vi "ProgInit.vi"(3 "error in (no error)":errorcluster, 4 "Intialize?":bool, 5 "EpiWrapper in":refnum<class "EpiWrapper.lvclass">) -> (0 "error out":errorcluster, 2 "EpiWrapper out":refnum<class "EpiWrapper.lvclass">)   [LabVIEW 2012, in "EpiWrapper.lvclass"]
uses:
  EpiWrapper.lvclass
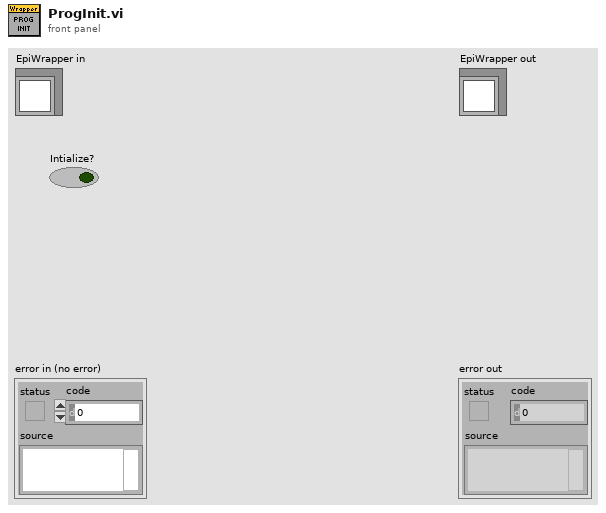
[diagram p1: front panel]
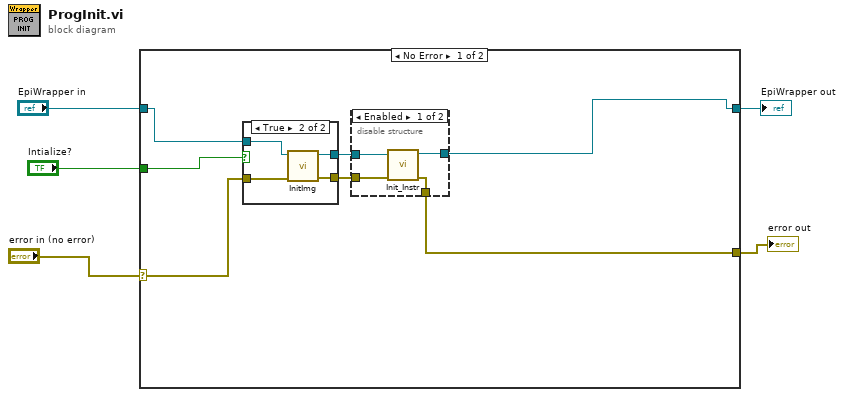
[diagram p0: block diagram]
diagram:
  n1 = case shown="No Error" "error in (no error)" {
    selector: "error in (no error)" -> [w6 w26]
    tunnel: [w9 w26] -> w4
    tunnel: [w10 w25] -> w2
    tunnel: "EpiWrapper in" -> [w7 w25]
    tunnel: "Intialize?" -> [w8 _]
    frame No Error {
      n2 = case shown="True" w8 {
        tunnel: [w14 w18] -> w12
        tunnel: [w13 w17] -> w11
        tunnel: w7 -> [w14 w16]
        tunnel: w6 -> [w13 w15]
        frame False {
        }
        frame True {
          n3 = call-dynamic "InitImg.vi"("error in (no error)"=w15, "EpiWrapper in"=w16) -> ("error out"=w17:errorcluster, "EpiWrapper out"=w18:refnum<class "EpiWrapper.lvclass">)  [unwired: 8 in]
        }
      }
      n4 = disable-structure shown="Enabled" {
        disable-tunnel: w12 -> [w22 w24]
        disable-tunnel: w11 -> [w21 w23]
        disable-tunnel: [w20 w24] -> w10
        disable-tunnel: [w19 w23] -> w9
        frame Enabled {
          n5 = call-dynamic "Init_Instr.vi"("error in (no error)"=w21, "EpiWrapper in"=w22) -> ("error out"=w19:errorcluster, "EpiWrapper out"=w20:refnum<class "EpiWrapper.lvclass">)  [unwired: 8 in]
        }
        frame Disabled {
        }
      }
    }
    frame Error {
    }
  }
  "error out" <- w4
  "EpiWrapper out" <- w2
